vi "SLIT_TRANS_Write_Config.vi"(4 "error in (no error)":errorcluster, 7 "Config Refnum":T1) -> (0 "error out":errorcluster, 3 "refnum out":T1)   [LabVIEW 2015]
uses:
  <vilib>/Utility/config.llb/Config Data RefNum.ctl
  GSP_SLIT_Global.vi
  <vilib>/Utility/config.llb/Write Key (I32).vi
  <vilib>/Utility/config.llb/NI_LVConfig.lvlib
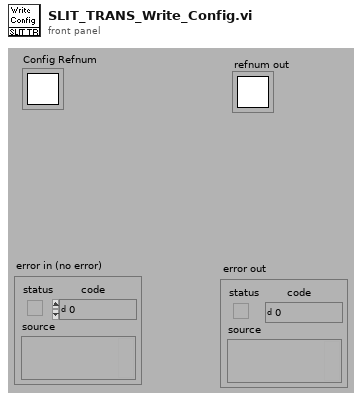
[diagram p1: front panel]
types:
  T1 = typedef "NI_LVConfig.lvlib/Config Data RefNum.ctl" = refnum<k1>
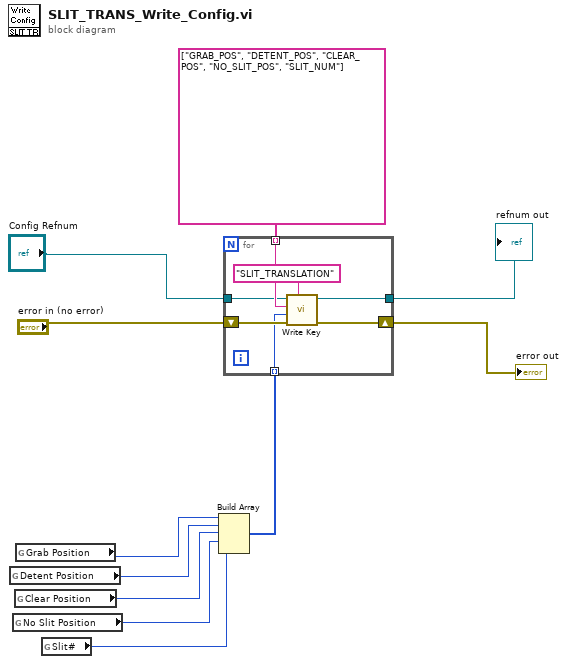
[diagram p0: block diagram]
diagram:
  n1 = global read "GSP_SLIT_Global.vi" "Detent Position"() -> (w4:i32)
  n2 = global read "GSP_SLIT_Global.vi" "No Slit Position"() -> (w2:i32)
  n3 = global read "GSP_SLIT_Global.vi" "Clear Position"() -> (w3:i32)
  n4 = global read "GSP_SLIT_Global.vi" "Grab Position"() -> (w5:i32)
  n5 = global read "GSP_SLIT_Global.vi" "Slit#"() -> (w1:i32)
  n6 = Build Array(w5, w4, w3, w2, w1) -> (w11:i32[])
  n7 = for {
    shift-right: [w16] -> w6
    shift-left: "error in (no error)" -> [w18]
    tunnel: [w15] -> w7
    tunnel: w11 -> [w12] mode=indexing
    tunnel: string[] ["GRAB_POS", "DETENT_POS", "CLEAR_POS", "NO_SLIT_POS", "SLIT_NUM"] -> [w14] mode=indexing
    tunnel: "Config Refnum" -> [w13]
    n8 = call-poly <vilib>:"Write Key.vi"("section"="SLIT_TRANSLATION", "error in (no error)"=w18, "value"=w12, "key"=w14, "refnum"=w13) -> ("error out"=w16:errorcluster, "refnum out"=w15:T1)  [unwired: 4 in, 1 out]
  }
  "error out" <- w6
  "refnum out" <- w7
